vi "checkUpperBound.vi"(8 "yStart in":i16, 9 "xStart in":i16, 10 "Y dimension":i16, 11 "X dimension":i16) -> (2 "yStart out":i16, 3 "xStart out":i16)   [LabVIEW 2015]
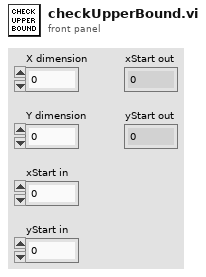
[diagram p1: front panel]
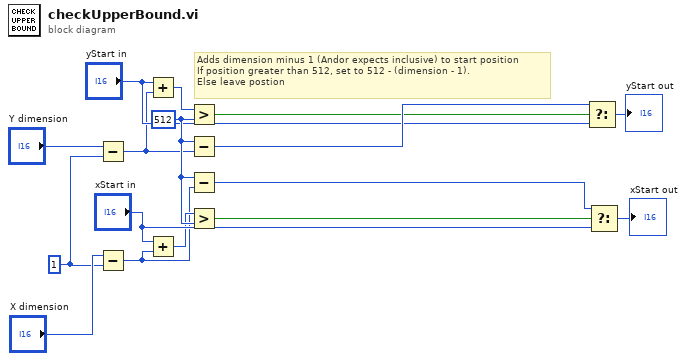
[diagram p0: block diagram]
diagram:
  w1 = i16 1 ("y")
  w14 = i16 512
  # "Adds dimension minus 1 (Andor expects inclusive) to start position\nIf position greater than 512, set to 512 - (dimension - 1).\nElse leave postion"
  n1 = Subtract(x="Y dimension", y=w1) -> (x-y=w2:i16)
  n2 = Subtract(x="X dimension", y=w1) -> (x-y=w4:i16)
  n3 = Add(x="yStart in", y=w2) -> (x+y=w7:i16)
  n4 = Add(x="xStart in", y=w4) -> (x+y=w6:i16)
  n5 = Greater?(x=w7, y=w14) -> (0:w8:bool)
  n6 = Subtract(x=w14, y=w2) -> (x-y=w13:i16)
  n7 = Subtract(x=w14, y=w4) -> (x-y=w12:i16)
  n8 = Greater?(x=w6, y=w14) -> (0:w9:bool)
  n9 = Select(t=w13, s=w8, f="yStart in") -> (s? t:f=→"yStart out":i16)
  n10 = Select(t=w12, s=w9, f="xStart in") -> (s? t:f=→"xStart out":i16)
